vi "VPI Set PWM Pulse.vi"(7 "pPulse":string, 9 "ChannelMask":u8, 10 "DevIndex":i32, 11 "DevType":i32) -> (3 "function return":i32, 5 "pPulse out":string)   [LabVIEW 2010, in "ControlPWM.lvlib"]
doc: "int WINAPI VPI_SetPWMPulse(int DevType, int DevIndex, unsigned char ChannelMask,unsigned char *pPulse);"
uses:
  ControlPWM.lvlib
  ControlPWM/Ginkgo_Driver.dll
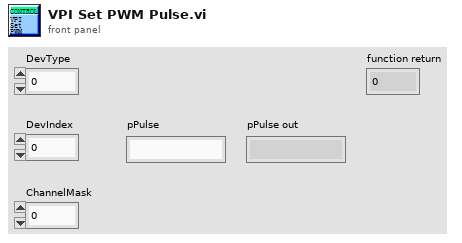
[diagram p1: front panel]
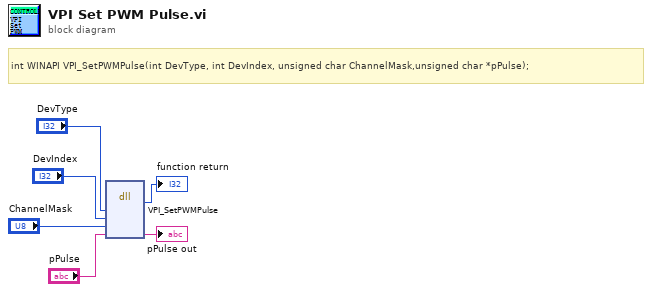
[diagram p0: block diagram]
diagram:
  # "int\tWINAPI VPI_SetPWMPulse(int DevType, int DevIndex, unsigned char ChannelMask,unsigned char *pPulse);"
  n1 = dll-call lib="E:/Project/vt_ginkgo/truck/Ginkgo Driver/vs2010/Ginkgo_USB-I2C&SPI&CAN_API_v2.0.3.3/lib/labview_32bit/ControlPWM/Ginkgo_Driver.*" fn="VPI_SetPWMPulse"("DevType"="DevType", "DevIndex"="DevIndex", "ChannelMask"="ChannelMask", "pPulse"="pPulse") -> (→"function return":i32, "pPulse"=→"pPulse out":string)  [unwired: 6 in, 2 out]
